vi "Handle Notification.vi"(8 "error in (no error)":errorcluster, 9 "Payload":string, 10 "Notification Type":string, 11 "Test Sequencer in":refnum<class "Test Sequencer.lvclass">) -> (0 "error out":errorcluster, 3 "Test Sequencer out":refnum<class "Test Sequencer.lvclass">)   [LabVIEW 2020, in "Test Sequencer.lvlib" / "Test Sequencer.lvclass"]
uses:
  Test Sequencer.lvclass
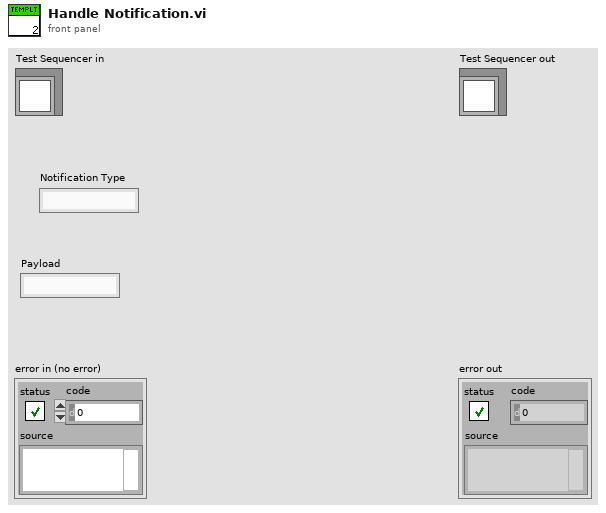
[diagram p1: front panel]
types:
  T1 = typedef "Params.ctl" = cluster{"Sequence Durations":dbl[], "Reset on Test Start":bool, "Current Sequence ID":u32, "Total Iterations":u32, "Last Timestamp":timestamp, "Number of Sequence Steps":i32}
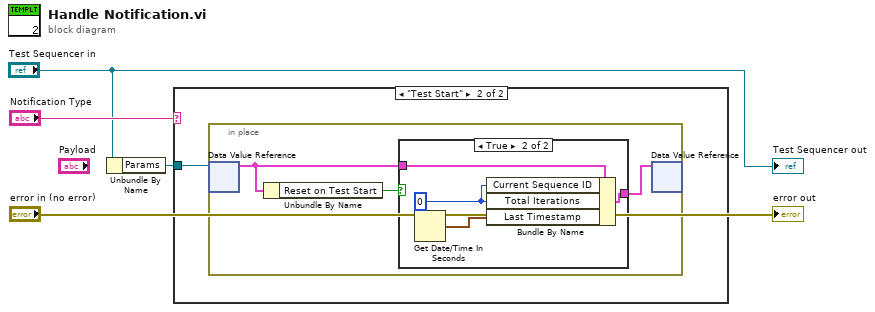
[diagram p0: block diagram]
diagram:
  n1 = Unbundle By Name("Test Sequencer in") -> ("Params"=w1:refnum<data-value>)
  n2 = case shown="\"Test Start\"" "Notification Type" {
    tunnel: w1 -> [_ w5]
    frame Default {
    }
    frame "Test Start" {
      n3 = in-place {
        n4 = in-place-dvr #1(w5) -> (w8:T1)  [unwired: 1 out]
        n5 = Unbundle By Name(w8) -> ("Reset on Test Start"=w7:bool)
        n6 = case shown="True" w7 {
          tunnel: w8 -> [w9 w13]
          tunnel: [w9 w12] -> w6
          frame False {
          }
          frame True {
            w11 = u32 0 ("Total Iterations")
            n7 = Get Date/Time In Seconds ("t0")() -> (seconds since 1Jan1904=w10:timestamp)
            n8 = Bundle By Name(cluster=w13, "Current Sequence ID"=w11, "Total Iterations"=w11, "Last Timestamp"=w10) -> (w12:T1)
          }
        }
        n9 = in-place-dvr #1(w6) -> ()  [unwired: 2 out]
      }
    }
  }
  "error out" <- "error in (no error)"
  "Test Sequencer out" <- "Test Sequencer in"
